vi "Unit 5 New.vi"() -> ()   [LabVIEW 2023]
panel:
  out "x < y?":bool
  out "Waveform Chart":cluster{"N текуща % ":dbl, "N2 % ":dbl}(graph)
  in  "к":dbl format="%#_13g"
  out "N след k минути":dbl format="%#_4g"
  out "Сумарно Време":dbl format="%#_2g"
  out "Сумарно \nВреме":dbl format="%#_4g"
  out "dN %/мин":dbl format="%#_1g"
  out "N след 1 минута":dbl format="%#_4g"
  out "Изминало време":dbl
  out "N текуща %":dbl format="%#_4g"
  in  "Режим":enum16{"=", "-", "+"}(ring)
  in  "dN/dT %/ h":dbl
  in  "N2 %":dbl
  in  "N1 % 1":dbl
  # "%"
  # "час"
  # "мин"
  # "%"
  # "мин"
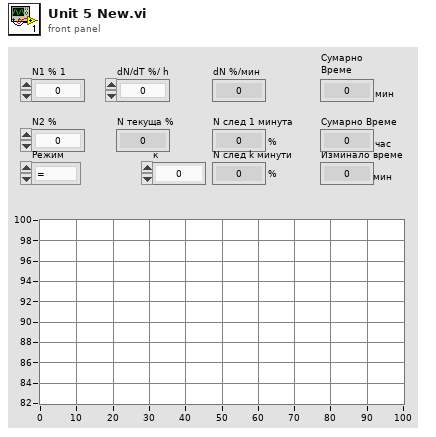
[diagram p1: front panel]
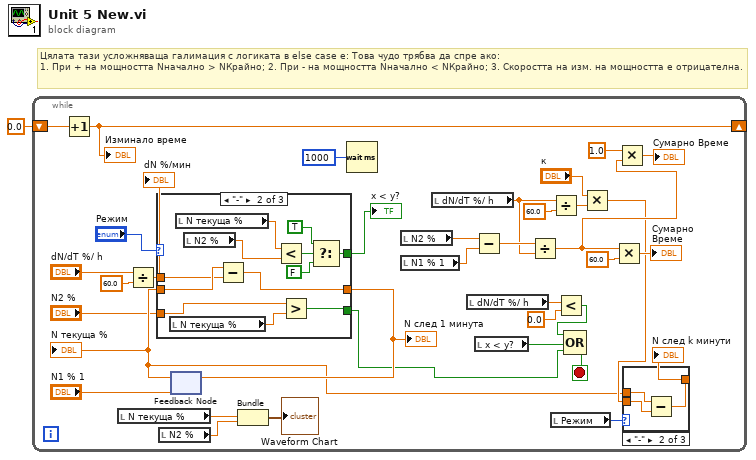
[diagram p0: block diagram]
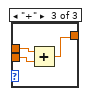
[diagram p3: hidden frame]
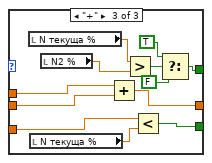
[diagram p5: hidden frame]
diagram:
  # "Цялата тази усложняваща галимация с логиката в else case e: Това чудо трябва да спре ако:\n1. При + на мощността Nначално > NКрайно; 2. При - на мощността Nначално < NКрайно; 3. Скоростта на изм. на мощността е отрицателна."
  n1 = while {
    shift-right: [w31] -> _
    shift-left: 0.0 -> [w33]
    stop <- w9 stop-if-true
    n2 = Increment(x=w33) -> (x+1=w31:dbl)
    "Изминало време" <- w31
    n3 = local read "N текуща %"() -> (w4:dbl)
    n4 = Divide(x="dN/dT %/ h", y=60.0) -> (x/y=w34:dbl)
    "dN %/мин" <- w34
    n5 = local read "N2 %"() -> (w3:dbl)
    n6 = feedback #1("N1 % 1") -> (w13:dbl)
    "N текуща %" <- w13
    n7 = case shown="\"-\"" "Режим" {
      tunnel: w13 -> [w45 w57 w69]
      tunnel: [w45 w56 w68] -> w18
      tunnel: w34 -> [_ w55 w67]
      tunnel: "N2 %" -> [_ w53 w65]
      tunnel: [_ w51 w64] -> w5
      tunnel: [_ w46 w58] -> w7
      frame "=", Default {
      }
      frame "-" {
        n8 = local read "N текуща %"() -> (w52:dbl)
        n9 = local read "N текуща %"() -> (w50:dbl)
        n10 = local read "N2 %"() -> (w54:dbl)
        n11 = Subtract(x=w57, y=w55) -> (x-y=w56:dbl)
        n12 = Less?(x=w50, y=w54) -> (x < y?=w49:bool)
        n13 = Greater?(x=w53, y=w52) -> (0:w51:bool)
        n14 = Select(t=TRUE, s=w49, f=FALSE) -> (s? t:f=w46:bool)
      }
      frame "+" {
        n15 = local read "N текуща %"() -> (w63:dbl)
        n16 = local read "N текуща %"() -> (w62:dbl)
        n17 = local read "N2 %"() -> (w66:dbl)
        n18 = Add(x=w67, y=w69) -> (x+y=w68:dbl)
        n19 = Greater?(x=w63, y=w66) -> (0:w61:bool)
        n20 = Less?(x=w65, y=w62) -> (x < y?=w64:bool)
        n21 = Select(t=TRUE, s=w61, f=FALSE) -> (s? t:f=w58:bool)
      }
    }
    "N след 1 минута" <- w18
    "x < y?" <- w7
    n22 = feedback-in #1(w18) -> ()
    n23 = Bundle("N текуща %"=w4, "N2 %"=w3) -> (→"Waveform Chart":cluster{"N текуща % ":dbl, "N2 % ":dbl})  [unwired: 1 in]
    n24 = Wait (ms)(milliseconds to wait=u32 1000) -> ()  [unwired: 1 out]
    n25 = local read "N2 %"() -> (w30:dbl)
    n26 = local read "N1 % 1"() -> (w29:dbl)
    n27 = local read "dN/dT %/ h"() -> (w16:dbl)
    n28 = local read "dN/dT %/ h"() -> (w12:dbl)
    n29 = Subtract(x=w30, y=w29) -> (x-y=w28:dbl)
    n30 = local read "x < y?"() -> (w6:bool)
    n31 = Divide(x=w28, y=w16) -> (x/y=w23:dbl)
    n32 = Divide(x=w16, y=60.0) -> (x/y=w17:dbl)
    n33 = local read "Режим"() -> (w19:enum16{"=", "-", "+"})
    n34 = Less?(x=w12, y=0.0) -> (x < y?=w10:bool)
    n35 = Compound Arithmetic op=OR(w10, w6, w5) -> (w9:bool)
    n36 = Multiply(x="к", y=w17) -> (x*y=w21:dbl)
    n37 = Multiply(x=w23, y=60.0) -> (x*y=→"Сумарно \nВреме":dbl)
    n38 = Multiply(x=1.0, y=w23) -> (x*y=→"Сумарно Време":dbl)
    n39 = case shown="\"-\"" w19 {
      tunnel: w21 -> [_ w41 w44]
      tunnel: [w38 w40 w43] -> w20
      tunnel: w13 -> [w38 w39 w42]
      frame "=", Default {
      }
      frame "-" {
        n40 = Subtract(x=w39, y=w41) -> (x-y=w40:dbl)
      }
      frame "+" {
        n41 = Add(x=w42, y=w44) -> (x+y=w43:dbl)
      }
    }
    "N след k минути" <- w20
  }
